vi "Retrieve Configuration Hash.vi"(8 "error in":errorcluster, 11 "Refnum in":T1) -> (0 "error out":errorcluster, 1 "Hash Good?":bool, 2 "Key Out":string, 3 "Refnum out":T1)   [LabVIEW 2013]
doc: "Check to see if the configuration file is valid. If the hash code that is in the configuration file does not match what we calculate, prompt the user to either call CAT for a valid one or to enter a code."
uses:
  <vilib>/Utility/config.llb/Config Data RefNum.ctl
  <vilib>/Utility/config.llb/Read Key (String).vi
  <vilib>/Utility/config.llb/Write Key (String).vi
  <vilib>/Utility/config.llb/NI_LVConfig.lvlib
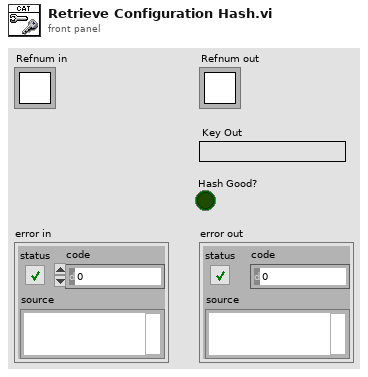
[diagram p1: front panel]
types:
  T1 = typedef "NI_LVConfig.lvlib/Config Data RefNum.ctl" = refnum<k1>
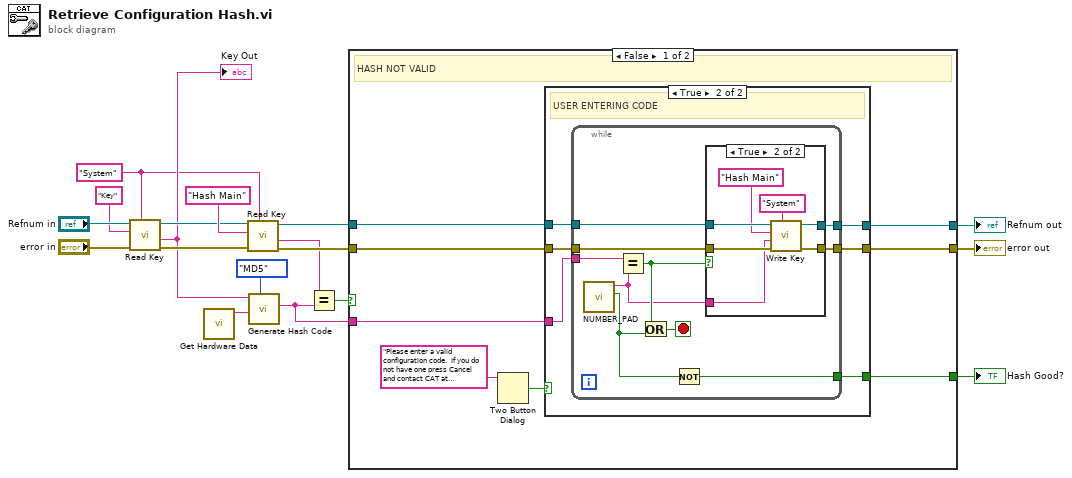
[diagram p0: block diagram]
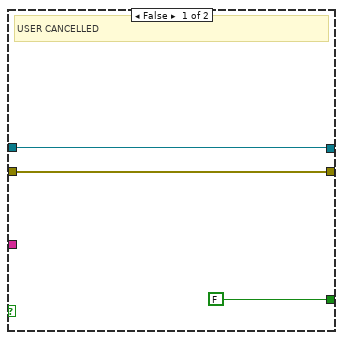
[diagram p2: hidden frame]
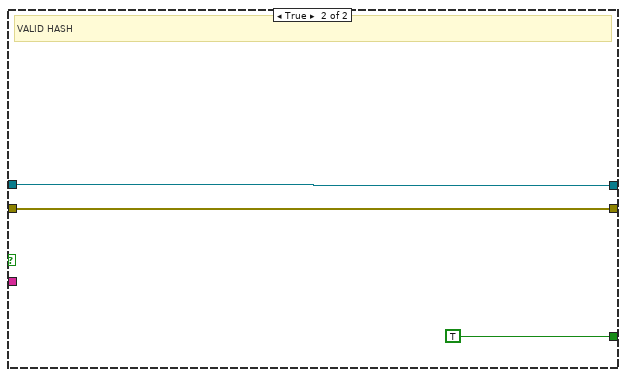
[diagram p4: hidden frame]
diagram:
  w1 = "System" ("section")
  n1 = call-poly <vilib>:"Read Key.vi"("section"=w1, "error in (no error)"="error in", "key"="Key", "refnum"="Refnum in") -> ("error out"=w8:errorcluster, "value"=w6:string, "refnum out"=w7:T1)  [unwired: 4 in, 1 out]
  "Key Out" <- w6
  n2 = call "Get Hardware Data.vi"() -> ("Fingerprint"=w14:string)  [unwired: 11 in]
  n3 = call-poly <vilib>:"Read Key.vi"("section"=w1, "error in (no error)"=w8, "key"="Hash Main", "refnum"=w7) -> ("error out"=w16:errorcluster, "value"=w10:string, "refnum out"=w15:T1)  [unwired: 4 in, 1 out]
  n4 = call "Generate Hash Code.vi"("Hash"=enum16{"MD5", "FNV-1"}."MD5", "Fingerprint"=w14, "Product ID"=w6) -> ("Hash"=w12:string)  [unwired: 7 in, 1 out]
  n5 = Equal?(x=w10, y=w12) -> (x = y?=w11:bool)
  n6 = case shown="False" w11 {
    tunnel: w12 -> [w19 _]
    tunnel: [w24 TRUE] -> w13
    tunnel: w15 -> [w23 w56]
    tunnel: w16 -> [w22 w55]
    tunnel: [w21 w56] -> w17
    tunnel: [w20 w55] -> w18
    frame False {
      # "HASH NOT VALID"
      n7 = Two Button Dialog(message="Please enter a valid configuration code.  If you do not have one press Cancel and contact CAT at  877-258-4883. ") -> (T button?=w25:bool)  [unwired: 2 in]
      n8 = case shown="True" w25 {
        tunnel: w19 -> [_ w35]
        tunnel: [FALSE w34] -> w24
        tunnel: w23 -> [w28 w33]
        tunnel: w22 -> [w27 w32]
        tunnel: [w28 w31] -> w21
        tunnel: [w27 w30] -> w20
        frame False {
          # "USER CANCELLED"
        }
        frame True {
          # "USER ENTERING CODE"
          n9 = while {
            tunnel: w35 -> [w45]
            tunnel: [w41] -> w34
            tunnel: w33 -> [w42]
            tunnel: w32 -> [w40]
            tunnel: [w38] -> w31
            tunnel: [w37] -> w30
            stop <- w43 stop-if-true
            n10 = call "NUMBER_PAD.vi"() -> ("Cancel?"=w44:bool, "number (out)"=w36:string)  [unwired: 10 in]
            n11 = Equal?(x=w45, y=w36) -> (x = y?=w39:bool)
            n12 = Or(x=w39, y=w44) -> (x .or. y?=w43:bool)
            n13 = Not(x=w44) -> (.not. x?=w41:bool)
            n14 = case shown="True" w39 {
              tunnel: w42 -> [w47 w54]
              tunnel: w40 -> [w46 w52]
              tunnel: [w47 w51] -> w38
              tunnel: [w46 w50] -> w37
              tunnel: w36 -> [_ w48]
              frame False {
              }
              frame True {
                n15 = call-poly <vilib>:"Write Key.vi"("section"="System", "error in (no error)"=w52, "value"=w48, "key"="Hash Main", "refnum"=w54) -> ("error out"=w50:errorcluster, "refnum out"=w51:T1)  [unwired: 4 in, 1 out]
              }
            }
          }
        }
      }
    }
    frame True {
      # "VALID HASH"
    }
  }
  "error out" <- w18
  "Refnum out" <- w17
  "Hash Good?" <- w13
